vi "User Help Update.vi"(8 "Error In":errorcluster, 10 "Enum":T1, 11 "User Help":string) -> (0 "Error Out":errorcluster, 3 "User Help Out":string)   [LabVIEW 2014]
doc: "Adds to the end of string enum constant as a string. Used to update user help."
uses:
  Controls/User Help.ctl
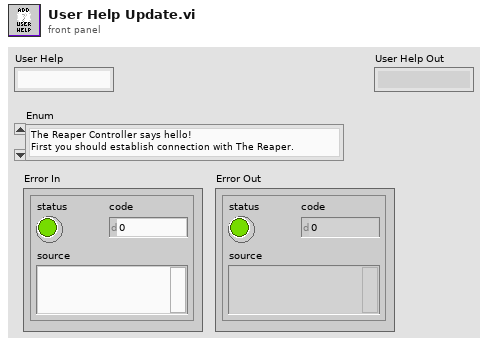
[diagram p1: front panel]
types:
  T1 = typedef "User Help.ctl" = enum16{"The Reaper Controller says hello!\nFirst you should establish connection with The Reaper.", "Connection established! Choose control mode.", "Something went wrong. Try another COM port.", "Disconnected. Do you want to connect again?", "Controls turned off", "Keyboard Mode", "Mouse Mode", "Pad Mode", "Autonomous Mode", "Unknown Operation occured", "Please connect before choosing control type!", "Settings available only if disconnected.", "Settings updated."}
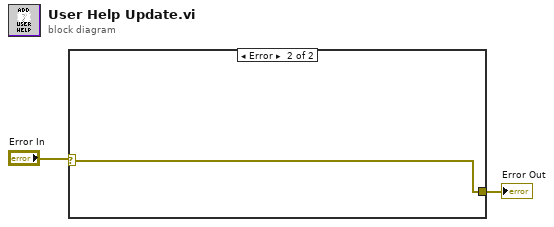
[diagram p0: block diagram]
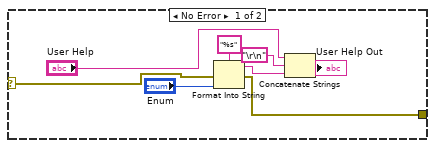
[diagram p2: hidden frame]
diagram:
  n1 = case shown="Error" "Error In" {
    selector: "Error In" -> [w4 w11]
    tunnel: [w3 w11] -> w1
    frame No Error {
      n2 = Format Into String(format string="%s", error in=w4, "Enum") -> (resulting string=w9:string, error out=w3:errorcluster)  [unwired: 1 in]
      n3 = Concatenate Strings("User Help", "\r\n", w9) -> (→"User Help Out":string)
    }
    frame Error {
    }
  }
  "Error Out" <- w1
